vi "UHR-Fleezers Control (host) - Lorentz v4.vi"() -> ()   [LabVIEW 2014] (continued)
                n2998 = call "move to saved stage position.vi"("Stage VISA resource name in"=w4451, "Position"=3, "Saved Stage Positions"=w4454) -> ("error out"=w4453:errorcluster)  [unwired: 1 in, 1 out]
                n2999 = local write "Stage Control Serial Error"(w4453) -> ()
              }
              frame #5 {
                w4456 = FALSE ("Stage Moving")
                n3000 = local write "Stage Moving"(w4456) -> ()
                n3001 = local write "AL Running"(w4456) -> ()
                n3002 = call <vilib>:"Beep.vi"() -> ()  [unwired: 3 in, 9 out]
              }
            }
          }
        }
      }
      event "Stop All": Value Change {
        n3003 = event-data() -> ()  [unwired: 7 out]
        n3004 = local read "Stop All"() -> (w4457:bool)
      }
    }
    n3005 = node-c288() -> ()  [unwired: 2 out]
  }
  n3006 = node-c288(w50) -> ()  [unwired: 1 out]
  n3007 = node-c288(w82) -> ()  [unwired: 1 out]
  n3008 = node-c288(w84) -> ()  [unwired: 1 out]
  n3009 = node-c288(w72) -> ()  [unwired: 1 out]
  n3010 = property on="Saved trap pos" class="WFGraph (strict)"("Visible"=FALSE) -> ()  [unwired: 2 in, 2 out]
  n3011 = property on="Trap Delta Graph" class="WFGraph (strict)"("Visible"=TRUE) -> ()  [unwired: 2 in, 2 out]
  n3012 = disable-structure shown="Disabled" {
    disable-tunnel: w75 -> [w4459 _]
    disable-tunnel: w74 -> [w4458 _]
    frame Disabled {
      n3013 = VISA Close(VISA resource name=w4459, error in (no error)=w4458) -> (error out=w4460:errorcluster)
      n3014 = call <vilib>:"Simple Error Handler.vi"("error in (no error)"=w4460) -> ()  [unwired: 1 in, 8 out]
    }
    frame Enabled {
    }
  }
  n3015 = disable-structure shown="Disabled" {
    disable-tunnel: [w4468 _] -> w36
    disable-tunnel: [w4464 _] -> w35
    disable-tunnel: [w4463 _] -> w34
    disable-tunnel: [w4462 _] -> w33
    disable-tunnel: [w4461 _] -> w32
    frame Disabled {
      # "n samples needed for data"
      n3016 = Unbundle By Name("sound format") -> ("sample rate (S/s)"=w4464:dbl)
      n3017 = call <vilib>:"Sound Output Configure.vi"("number of samples/ch"="number of samples/ch", "sample mode"="sample mode", "sound format"="sound format", "device ID"="device ID") -> ("task ID"=w4468:T60)  [unwired: 6 in, 1 out]
      n3018 = local read "DMA Update Period (s)"() -> (w4465:dbl)
      n3019 = Multiply(x=w4465, y=w4464) -> (x*y=w4463:dbl)
      n3020 = for "Sound time base" {
        N: w4463 -> [_]
        tunnel: [w4472] -> w4466 mode=indexing
        i -> [w4472]
      }
      n3021 = Reciprocal(x=w4464) -> (1/x=w4462:dbl)
      n3022 = Multiply(x=w4466, y=w4462) -> (x*y=w4461:dbl[])
    }
    frame Enabled {
    }
  }
  n3023 = timed-loop "Main data acquisition loop (get data, process data for display, and save data to disk)" {
    tunnel: w31 -> [w4562]
    tunnel: w44 -> [w4561]
    tunnel: [w4821] -> w96
    tunnel: [w4816] -> w95
    timing: w89 -> [_]
    timing-out: [_] -> w88
    tunnel: w66 -> [w4728]
    tunnel: [w4618] -> w37
    tunnel: w36 -> [w4617]
    tunnel: w35 -> [w4615]
    tunnel: w34 -> [w4614]
    tunnel: w33 -> [w4613]
    tunnel: w32 -> [w4612]
    tunnel: w21 -> [w4553]
    tunnel: w20 -> [w4552]
    tunnel: [w4547] -> w19
    stop <- "Stop All" stop-if-true
    w4492 = 2.0
    w4518 = 3276.7
    w4675 = "Initialize"
    # "Cursor control of MCL trap position"
    # "Values for plotting"
    # "Added by Ronen - the limits imposed on amplitudes sent to AOM\nare not explicitly imposed when using intensity feedback. At amplitude of \n~48% FB intensity is ~1.8, if while feedback is on the value passes 1.8, feedback\nis turned off (indication that feedback algorithm overshoots)."
    # "List of channels in order (X or Y only):\nT1 X (mV)\nT2 X (mV)\nT1 X (nm)\nT2 X (nm)\nT1 FX (pN)\nT2 FX (pN)\nPosition Difference (nm)\nAPD1\nAPD2\nAPD3"
    # "T2 sum"
    # "T1 sum"
    n3024 = node-c288() -> ()  [unwired: 2 out]
    n3025 = First Call?() -> (First Call?: T/F=w4688:bool)
    n3026 = Or(x="Reset", y=w4688) -> (x .or. y?=w4689:bool)
    n3027 = Or(x="Start AOD Scan", y="Trap Raster Scan") -> (x .or. y?=w4775:bool)
    n3028 = case "Reset data stream (manual reset or at begining of some rastering and imaging)" shown="True" w4689 {
      tunnel: w4562 -> [w5574 w5582]
      tunnel: w4561 -> [w5573 w5581]
      tunnel: [w5574 w5576] -> w4592
      tunnel: [w5573 w5575] -> w4593
      frame False {
      }
      frame True {
        w5579 = TRUE ("AI to FIFO")
        n3029 = call "reset FPGA DMA.vi"("error in"=w5581, "FPGA VI Reference In"=w5582) -> ("error out"=w5577:errorcluster, "FPGA VI Reference Out"=w5578:T50)
        n3030 = local write "Overflow (data lost)"(FALSE ("Overflow (data lost)")) -> ()
        n3031 = xnode "Read/Write Control"("FPGA VI Reference In"=w5578, "error in"=w5577, "AI to FIFO"=w5579, "APD to FIFO"=w5579) -> ("FPGA VI Reference Out"=w5576:T50, "error out"=w5575:errorcluster)
      }
    }
    n3032 = case "Start active calibration (oscillate traps precisely)" shown="True" "Active Cal" {
      tunnel: w4593 -> [w4924 w4932]
      tunnel: w4592 -> [w4923 w4933]
      tunnel: [w4924 w4929] -> w4591
      tunnel: [w4923 w4930] -> w4590
      frame False {
      }
      frame True {
        w4925 = TRUE ("APD to FIFO")
        n3033 = call "reset FPGA DMA.vi"("error in"=w4932, "FPGA VI Reference In"=w4933) -> ("error out"=w4926:errorcluster, "FPGA VI Reference Out"=w4927:T50)
        n3034 = local write "Active Cal"(FALSE ("Active Cal")) -> ()
        n3035 = local write "Save Calibration"(TRUE ("Save Calibration")) -> ()
        n3036 = xnode "Read/Write Control"("FPGA VI Reference In"=w4927, "error in"=w4926, "AI to FIFO"=w4925, "APD to FIFO"=w4925) -> ("FPGA VI Reference Out"=w4930:T50, "error out"=w4929:errorcluster)
      }
    }
    n3037 = case shown="True" "Read Lateness and Rel Phase" {
      tunnel: w4562 -> [w5148 w5179]
      tunnel: w4561 -> [w5149 w5178]
      tunnel: [w5148 w5150] -> w4514
      tunnel: [w5149 w5151] -> w4764
      frame False {
      }
      frame True {
        n3038 = xnode "Read/Write Control"("FPGA VI Reference In"=w5179, "error in"=w5178) -> ("FPGA VI Reference Out"=w5150:T50, "error out"=w5151:errorcluster, "GI Relative phase"=→"GI relative phase":i16, "Relative phase"=→"Relative phase (AI1)":i16, "AI Late Counter"=→"Late Counter (AI1)":u8, "GI Late Counter"=→"GI Late Counter":u8, "MCL Late Counter"=→"MCL Late Counter":u8, "MCL Relative Phase"=→"Relative Phase (MCL)":i16, "APD Acq Relative Phase"=→"APD Acq Relative Phase":i16, "APD 1 Gate Relative Phase"=→"APD 1 Gate Relative Phase":i16, "APD 2 Gate Relative Phase"=→"APD 2 Gate Relative Phase":i16, "APD Acq Late Counter"=→"APD Acq Late Counter":u8, "APD 1 Gate Late Counter"=→"APD 1 Gate Late Counter":u8, "APD 2 Gate Late Counter"=→"APD 2 Gate Late Counter":u8, "Green FB Relative Phase"=→"Relative phase (Green FB)":i16, "GI Relative phase 2"=→"GI relative phase 2":i16, "GI Late Counter 2"=→"GI Late Counter 2":u8, "Trap Pos FIFO Timeout"=→"Trap Pos FIFO Timeout":u16, "Trap AI FIFO Timeout"=→"Trap AI FIFO Timeout":u16, "RI Late Counter"=→"RI Late Counter":u8, "RI Relative phase"=→"RI relative phase":i16, "Green Late Counter"=→"Green AI Late Counter":u8, "BI Late Counter (AO)"=→"Late Counter (BI AO)":u8, "Blue Late Counter (D)"=→"Late Counter (BI DO)":u8, "BI Relative phase (AO)"=→"Relative phase (BI AO)":i16, "BI Relative phase (D)"=→"Relative phase (BI DO)":i16, "APD 3 Gate Late Counter"=→"APD 3 Gate Late Counter":u8, "APD 3 Gate Relative Phase"=→"APD 3 Gate Relative Phase":i16)
      }
    }
    n3039 = Compound Arithmetic op=OR("Start MCL Scan", "Confocal Image", "Confocal Linescan") -> (w4560:bool)
    n3040 = And(x="Save Data (MCL)", y=w4560) -> (x .and. y?=w4794:bool)
    n3041 = case "Start AOM raster scan" shown="True" w4775 {
      tunnel: w4590 -> [w5433 w5443]
      tunnel: w4591 -> [w5432 w5442]
      tunnel: [w5433 w5436] -> w4797
      tunnel: [w5432 w5435] -> w4796
      frame False {
      }
      frame True {
        n3042 = case shown="True" "Restart DMA? (AOD)" {
          tunnel: [w5472 w5474] -> w5437
          tunnel: [w5471 w5473] -> w5438
          tunnel: w5443 -> [w5472 w5476]
          tunnel: w5442 -> [w5471 w5475]
          frame False {
          }
          frame True {
            n3043 = local write "Overflow (data lost)"(FALSE ("Overflow (data lost)")) -> ()
            n3044 = call "reset FPGA DMA.vi"("error in"=w5475, "FPGA VI Reference In"=w5476) -> ("error out"=w5473:errorcluster, "FPGA VI Reference Out"=w5474:T50)
          }
        }
        n3045 = local write "Trap Raster Scan"(FALSE ("Trap Raster Scan")) -> ()
        n3046 = case shown="True" "Move MCL Also?" {
          tunnel: w5438 -> [w5446 w5466]
          tunnel: w5437 -> [w5447 w5467]
          tunnel: [w5445 w5470] -> w5436
          tunnel: [w5444 w5469] -> w5435
          frame False {
            w5448 = TRUE ("AI to FIFO")
            n3047 = xnode "Read/Write Control"("FPGA VI Reference In"=w5447, "error in"=w5446, "AI to FIFO"=w5448, "APD to FIFO"=w5448, "Start scan"=w5448) -> ("FPGA VI Reference Out"=w5445:T50, "error out"=w5444:errorcluster)
          }
          frame True {
            w5464 = FALSE ("1D or 2D Scan?")
            w5468 = TRUE ("AI to FIFO")
            n3048 = local read "Scan Range (nm)"() -> (w5461:dbl)
            n3049 = local read "Scan steps (AOD)"() -> (w5455:u64)
            n3050 = local read "Total Counts (ticks)"() -> (w5456:u16)
            n3051 = local read "Cycles/step (AOD)"() -> (w5454:u64)
            n3052 = local read "Number of F/B Scans (AOD)"() -> (w5463:u16)
            n3053 = Bundle("Scan Range (nm)"=w5461, "MCL Step Position Ratio"="MCL Step Position Ratio", "MCL/AOM Scale Tweak"="MCL/AOM Scale Tweak", "MCL X Cal (nm/V)"="MCL X Cal (nm/V)", "MCL Step Increment (V_int)"="MCL Step Increment (V_int)", "Total Counts (ticks)"=w5456, "Scan steps (AOD)"=w5455, "Cycles/step (AOD)"=w5454) -> (w5453:T67)  [unwired: 1 in]
            n3054 = call "Calculate MCL scan parameters.vi"("Input parameters"=w5453) -> ("Scan steps(MCL)"=w5452:dbl, "Scan Freq. Increment (MCL)"=w5451:dbl, "MCL Count"=w5450:dbl)
            "MCL Count" <- w5450
            n3055 = xnode "Read/Write Control"("FPGA VI Reference In"=w5467, "error in"=w5466, "Scan steps (MCL)"=w5452, "Number of scans (MCL)"=w5463, "Cycles per step (MCL)"=u64 1, "Scan freq.  increment (MCL)"=w5451, "1D or 2D Scan?"=w5464, "MCL Scan Axis"=w5464, "Cont. Scan (MCL)"=w5464, "MCL count"=w5450) -> ("FPGA VI Reference Out"=w5449:T50, "error out"=w5465:errorcluster)
            n3056 = local write "MCL Scanning"(w5468) -> ()
            n3057 = local write "wait to reset values"(w5468) -> ()
            n3058 = xnode "Read/Write Control"("FPGA VI Reference In"=w5449, "error in"=w5465, "AI to FIFO"=w5468, "APD to FIFO"=w5468, "Start scan"=w5468, "Start scan (MCL)"=w5468) -> ("FPGA VI Reference Out"=w5470:T50, "error out"=w5469:errorcluster)
          }
        }
        "Raster Scanning..." <- TRUE ("Scanning...")
      }
    }
    n3059 = case "Start MCL raster scan" shown="True" w4560 {
      tunnel: w4797 -> [w5361 w5376]
      tunnel: w4796 -> [w5360 w5375]
      tunnel: [w5361 w5371] -> w4727
      tunnel: [w5360 w5370] -> w4726
      tunnel: [FALSE w5369] -> w4780
      tunnel: "Start MCL Scan" -> [_ w5364]
      tunnel: "Confocal Image" -> [_ w5363]
      tunnel: "Confocal Linescan" -> [_ _]
      frame False {
      }
      frame True {
        w5369 = TRUE
        n3060 = case shown="True" "Restart DMA? (MCL)" {
          tunnel: [w5405 w5407] -> w5374
          tunnel: [w5404 w5406] -> w5373
          tunnel: w5376 -> [w5405 w5410]
          tunnel: w5375 -> [w5404 w5409]
          frame False {
          }
          frame True {
            n3061 = call "reset FPGA DMA.vi"("error in"=w5409, "FPGA VI Reference In"=w5410) -> ("error out"=w5406:errorcluster, "FPGA VI Reference Out"=w5407:T50)
            n3062 = local write "Overflow (data lost)"(FALSE ("Overflow (data lost)")) -> ()
          }
        }
        n3063 = case shown="False" w5364 {
          tunnel: w5363 -> [w5379 _]
          frame False {
            n3064 = property on="Confocal Image" class="Bool (strict)"("Value"=FALSE ("Start Confocal Map")) -> ()  [unwired: 2 in, 2 out]
            n3065 = property on="2D or 1D Scan" class="Bool (strict)"("Val(Sgnl)"=w5379) -> ()  [unwired: 2 in, 2 out]
          }
          frame True {
          }
        }
        n3066 = local write "Tab Control 6"(T4."Imaging" ("Tab Control 6")) -> ()
        n3067 = local write "MCL Scanning"(w5369) -> ()
        n3068 = local read "AO2"() -> (w5365:dbl)
        n3069 = local read "AO1"() -> (w5366:dbl)
        n3070 = case shown="True" "Center Scan" {
          tunnel: w5374 -> [w5386 w5403]
          tunnel: w5373 -> [w5385 w5402]
          tunnel: [w5384 w5401] -> w5371
          tunnel: [w5383 w5400] -> w5370
          tunnel: [w5381 w5388] -> w5368
          tunnel: [w5380 w5387] -> w5367
          tunnel: w5366 -> [w5381 w5393]
          tunnel: w5365 -> [w5380 w5392]
          frame False {
            w5382 = TRUE ("AI to FIFO")
            n3071 = xnode "Read/Write Control"("FPGA VI Reference In"=w5386, "error in"=w5385, "AI to FIFO"=w5382, "APD to FIFO"=w5382, "Start scan (MCL)"=w5382) -> ("FPGA VI Reference Out"=w5384:T50, "error out"=w5383:errorcluster)
          }
          frame True {
            w5399 = TRUE ("AI to FIFO")
            n3072 = local read "Actual MCL Inc (V)"() -> (w5396:dbl)
            n3073 = local read "Scan steps (MCL)"() -> (w5395:u64)
            n3074 = local read "Scan lines (y)"() -> (w5394:u64)
            n3075 = local read "2D or 1D Scan"() -> (w5389:bool)
            n3076 = local read "Fast Scan Dir"() -> (w5390:bool)
            n3077 = Bundle("Actual MCL Inc (V)"=w5396, "Scan steps (MCL)"=w5395, "Scan lines (y)"=w5394, "AO1"=w5393, "AO2"=w5392) -> (w5391:T68)  [unwired: 1 in]
            n3078 = call "Center Scan calculation.vi"("2D or 1D Scan"=w5389, "Fast Scan Dir"=w5390, "Input parameters"=w5391) -> ("AO2"=w5387:dbl, "AO1"=w5388:dbl)
            n3079 = call "Volt to I16.vi"("Voltage In"=w5388) -> ("I16 Voltage Out"=w5398:i16)
            n3080 = call "Volt to I16.vi"("Voltage In"=w5387) -> ("I16 Voltage Out"=w5397:i16)
            n3081 = xnode "Read/Write Control"("FPGA VI Reference In"=w5403, "error in"=w5402, "AI to FIFO"=w5399, "APD to FIFO"=w5399, "Start scan (MCL)"=w5399, "AO1"=w5398, "AO2"=w5397) -> ("FPGA VI Reference Out"=w5401:T50, "error out"=w5400:errorcluster)
          }
        }
        "Initial Y" <- w5368
        "Initial X" <- w5367
        "wait to reset values" <- w5369
      }
    }
    n3082 = xnode "Read/Write Control"("FPGA VI Reference In"=w4514) -> ("FPGA VI Reference Out"=w4473:T50, "BD1 Frequency Out 1"=w4516:u64)  [unwired: 1 in, 1 out]
    n3083 = And(x="Save scans", y=w4775) -> (x .and. y?=w4795:bool)
    n3084 = call "IR AOM word to freq.vi"("Frequency Word In (U64)"=w4516) -> ("Frequency Out (MHz)"=w4515:dbl)
    n3085 = local read "BD 1 Frequency 2 (MHz)"() -> (w4575:dbl)
    n3086 = Subtract(x=w4575, y=w4515) -> (x-y=w4568:dbl)
    "Current deltaF (MHz)" <- w4568
    n3087 = control-ref of="Piezo trap cursor control"() -> (w4474:refnum<vi>)
    n3088 = Unbundle By Name("Cursor control") -> ("X"=w4476:bool, "Y"=w4475:bool)
    n3089 = local read "APD Elements/DMA read"() -> (w4632:u32)
    n3090 = local read "Trap AI Elements/DMA read"() -> (w4762:u32)
    n3091 = case shown="False" w4476 {
      tunnel: w4474 -> [w4848 w4858]
      tunnel: w4473 -> [_ w4850]
      frame False {
        n3092 = local read "T3 X (V)"() -> (w4849:dbl)
        n3093 = property class="XYGraph (strict)"(reference=w4848, "Cursor.Cursor X"=w4849) -> ()  [unwired: 1 in, 2 out]
      }
      frame True {
        n3094 = property class="XYGraph (strict)"(reference=w4858) -> ("Cursor.Cursor X"=w4855:dbl)  [unwired: 1 in, 2 out]
        n3095 = In Range and Coerce(upper limit=10.0, x=w4855, lower limit=0.0) -> (coerced(x)=w4853:dbl)  [unwired: 1 out]
        n3096 = Multiply(x=3276.7, y=w4853) -> (x*y=w4852:dbl)
        n3097 = To Unsigned Word Integer(number=w4852) -> (unsigned 16bit integer=w4851:u16)
        n3098 = xnode "Read/Write Control"("FPGA VI Reference In"=w4850, "Piezo Trap X (AO5)"=w4851) -> ()  [unwired: 1 in, 2 out]
      }
    }
    n3099 = case shown="False" w4475 {
      tunnel: w4474 -> [w4835 w4847]
      tunnel: w4473 -> [_ w4838]
      frame False {
        n3100 = local read "T3 Y (V)"() -> (w4837:dbl)
        n3101 = Negate(x=w4837) -> (-x=w4836:dbl)
        n3102 = property class="XYGraph (strict)"(reference=w4835, "Cursor.Cursor Y"=w4836) -> ()  [unwired: 1 in, 2 out]
      }
      frame True {
        n3103 = property class="XYGraph (strict)"(reference=w4847) -> ("Cursor.Cursor Y"=w4844:dbl)  [unwired: 1 in, 2 out]
        n3104 = In Range and Coerce(upper limit=0.0, x=w4844, lower limit=-10.0) -> (coerced(x)=w4843:dbl)  [unwired: 1 out]
        n3105 = Negate(x=w4843) -> (-x=w4841:dbl)
        n3106 = Multiply(x=3276.7, y=w4841) -> (x*y=w4840:dbl)
        n3107 = To Unsigned Word Integer(number=w4840) -> (unsigned 16bit integer=w4839:u16)
        n3108 = xnode "Read/Write Control"("FPGA VI Reference In"=w4838, "Piezo Trap Y (AO4)"=w4839) -> ()  [unwired: 1 in, 2 out]
      }
    }
    n3109 = local read "Trap Pos Elements/DMA read"() -> (w4723:u32)
    n3110 = local read "DMA Update Period (s)"() -> (w4550:dbl)
    n3111 = xnode "Invoke Method"("FPGA VI Reference In"=w4727, "error in"=w4726, "Number of Elements"=w4723, "Timeout (ms)"=-1) -> ("Data"=w4695:u16[], "Elements Remaining"=→"Trap Pos FIFO El Remaining":u32)  [unwired: 2 out]
    n3112 = xnode "Get Trap Data"("FPGA VI Reference In"=w4727, "error in"=w4726, "Number of Elements"=w4762, "Timeout (ms)"=-1 ("Timeout")) -> ("FPGA VI Reference Out"=w4574:T50, "error out"=w4665:errorcluster, "Data"=w4557:i16[], "Elements Remaining"=w4829:u32)
    "FIFO El. Rem." <- w4829
    n3113 = local read "Trap AI FIFO Depth"() -> (w4831:u32)
    n3114 = xnode "Get APD Data"("FPGA VI Reference In"=w4727, "error in"=w4726, "Number of Elements"=w4632, "Timeout (ms)"=-1) -> ("Data"=w4529:u32[], "Elements Remaining"=→"APD FIFO Elements Remaining":u32)  [unwired: 2 out]
    n3115 = feedback #1(0.0) -> (w4718:dbl)
    n3116 = To Time Stamp(1:w4718) -> (0:w4512:timestamp)
    n3117 = Add(x=w4550, y=w4718) -> (x+y=w4806:dbl)
    n3118 = feedback-in #1(w4806) -> ()
    n3119 = Subtract(x=w4831, y=w4762) -> (x-y=w4830:u32)
    n3120 = local read "APD Integration Time (s)"() -> (w4521:dbl)
    n3121 = Divide(x=w4829, y=w4830) -> (x/y=w4828:dbl)
    "Buffer Status" <- w4828
    n3122 = local read "Trap Sets"() -> (w4558:u32)
    n3123 = Divide(x=w4550, y="PSD Data Period (s)") -> (x/y=w4549:dbl)
    n3124 = Equal?(x=w4828, y=1.0) -> (x = y?=w4826:bool)
    n3125 = local read "Number of APDs"() -> (w4528:u8)
    n3126 = Decimate 1D Array(w4695) -> (w4692:u16[], w4694:u16[], w4693:u16[], w4519:u16[], w4517:u16[])
    n3127 = To Unsigned Long Integer(number=w4549) -> (unsigned 32bit integer=w4548:u32)
    n3128 = case "Alert buffer overflow" shown="True" w4826 {
      frame False {
      }
      frame True {
        n3129 = call <vilib>:"Beep.vi"() -> ()  [unwired: 3 in, 9 out]
        "Overflow (data lost)" <- TRUE ("Overflow (data lost)")
      }
    }
    n3130 = To Unsigned Long Integer(number=w4692) -> (unsigned 32bit integer=w4691:u32[])
    n3131 = Join Numbers(hi=w4694, lo=w4693) -> ((hi.lo)=w4690:u32[])
    n3132 = Divide(x=w4519, y=w4518) -> (x/y=w4500:dbl[])
    n3133 = Divide(x=w4517, y=w4518) -> (x/y=w4499:dbl[])
    n3134 = call "Arduino input-output.vi"("VISA resource name"=w4553, "Sets to read"=w4548, "Error in"=w4552) -> ("VISA resource out"=w4547:refnum<visa-resource-name>, "Channel names"=w4537:string[], "Output"=w4536:dbl[][], "Error out"=→"Serial Error out":errorcluster)
    n3135 = call "deinterlace.vi"("Detector type"="Detector Type", "Data"=w4557, "Trap sets"=w4558, "Flip x sign"="Flip X Sign") -> ("Channel pattern"=w4554:i32, "Channel names"=w4533:string[], "Deinterlaced normalized data"=w4534:dbl[][], "Deinterlaced data"=w4555:i16[])
    n3136 = Join Numbers(hi=w4691, lo=w4690) -> ((hi.lo)=w4685:u64[])
    n3137 = local read "Data Period (s)"() -> (w4506:dbl)
    n3138 = call "APD data extraction.vi"("Data"=w4529, "Number of APD's"=w4528, "APD integration time (s)"=w4521, "APD Ave N"="APD Ave N", "APD Disp. Downsample"="APD Disp. Downsample", "APD Disp. Scale"="APD Disp. Scale", "Time Stamp"=w4512) -> ("Output cluster"=→"APD rates cluster":T2, "Output Data"=w4524:T69, "Output waveform"=w4523:waveform(dbl)[], "APD Display period (s)"=w4522:dbl)
    "APD Display Period (s)" <- w4522
    n3139 = call "IR AOM word to freq - vec.vi"("Frequency Word In (double vec)"=w4685) -> ("Frequency Out"=w4722:dbl[])
    n3140 = Decimate 1D Array(w4499) -> (w4496:dbl[], w4495:dbl[])
    n3141 = Decimate 1D Array(w4500) -> (w4498:dbl[], w4497:dbl[])
    n3142 = Add(x=w4498, y=w4497) -> (x+y=w4494:dbl[])
    n3143 = Add(x=w4496, y=w4495) -> (x+y=w4493:dbl[])
    n3144 = Decimate 1D Array(w4722) -> (w4721:dbl[], w4720:dbl[])
    n3145 = Divide(x=w4494, y=w4492) -> (x/y=w4490:dbl[])
    n3146 = Divide(x=w4493, y=w4492) -> (x/y=w4491:dbl[])
    n3147 = Reciprocal(x=w4522) -> (1/x=→"APD Display Freq. (Hz)":dbl)
    n3148 = call "Generate Waveform.vi"("Downsampling"="PSD downsample", "Data Period (s)"="PSD Data Period (s)", "Data"=w4536, "Plot names"=w4537, "Time Stamp"=w4512) -> ("Downsampled data"=w4535:waveform(dbl)[])  [unwired: 1 out]
    n3149 = Build Array(w4721, w4720, w4490, w4491) -> (w4513:dbl[][])
    n3150 = for {
      tunnel: w4536 -> [w4874] mode=indexing
      tunnel: [w4873] -> w4543 mode=indexing
      n3151 = call-poly <vilib>:"Mean.vi"("X"=w4874) -> ("mean"=w4873:dbl)  [unwired: 1 out]
    }
    n3152 = Multiply(x=w4506, y="Trap Disp. Downsample") -> (x*y=w4719:dbl)
    "Display Period (s)" <- w4719
    n3153 = for {
      tunnel: w4534 -> [w4876] mode=indexing
      tunnel: [w4875] -> w4542 mode=indexing
      n3154 = call-poly <vilib>:"Mean.vi"("X"=w4876) -> ("mean"=w4875:dbl)  [unwired: 1 out]
    }
    n3155 = call "Generate Waveform.vi"("Downsampling"="Trap Disp. Downsample", "Data Period (s)"=w4506, "Data"=w4534, "Plot names"=w4533, "Time Stamp"=w4512) -> ("Downsampled data"=w4531:waveform(dbl)[], "Non downsampled waveform"=w4530:waveform(dbl)[])
    n3156 = Multiply(x="APD Disp. Scale", y=w4523) -> (x*y=w4740:waveform(dbl)[])
    n3157 = Reciprocal(x=w4719) -> (1/x=→"Trap Disp. Freq. (Hz)":dbl)
    n3158 = Insert Into Array(array=w4543, index=0, new element=w4542) -> (→"Values":dbl[])
    n3159 = Multiply(x="APD Disp. Downsample", y=w4521) -> (x*y=w4739:dbl)
    n3160 = Decimate 1D Array(w4555) -> (w4710:i16[], w4709:i16[], w4707:i16[], w4706:i16[])  [unwired: 9 out]
    n3161 = Divide(x=w4740, y=w4739) -> (x/y=w4637:waveform(dbl)[])
    n3162 = Insert Into Array(array=w4537, index=0, new element=w4533) -> (→"AI labels":string[])
    n3163 = case shown="1" "Plot Trap Positions" {
      tunnel: [w4859 w4868] -> w4507
      frame 0, Default {
        n3164 = local read "BD 1 Frequency 2 (MHz)"() -> (w4862:dbl)
        n3165 = local read "BD 1 Frequency 1 (MHz)"() -> (w4863:dbl)
        n3166 = local read "T3 Y (V)"() -> (w4860:dbl)
        n3167 = local read "T3 X (V)"() -> (w4861:dbl)
        n3168 = Build Array(w4863, w4862, w4861, w4860) -> (w4859:dbl[])
      }
      frame 1 {
        w4867 = 75.0
        n3169 = Unbundle By Name("Piezo trap 0 position relative to 75 MHz") -> ("X (V)"=w4865:dbl, "Y (V)"=w4864:dbl)
        n3170 = Build Array(w4867, w4867, w4865, w4864) -> (w4868:dbl[])
      }
    }
    n3171 = Divide(x=w4710, y=w4709) -> (x/y=w4711:dbl[])
    n3172 = Divide(x=w4707, y=w4706) -> (x/y=w4708:dbl[])
    n3173 = local read "AOM X Cal (nm/MHz)"() -> (w4509:dbl)
    n3174 = Split 1D Array(array=w4711, index="N El. to Ave.") -> (second subarray=w4714:dbl[])  [unwired: 1 out]
    n3175 = Split 1D Array(array=w4708, index="N El. to Ave.") -> (second subarray=w4713:dbl[])  [unwired: 1 out]
    n3176 = Index Array(array=w4637, index=0) -> (element=w4735:waveform(dbl))
    n3177 = Index Array(array=w4637, index=1) -> (element=w4733:waveform(dbl))
    n3178 = Index Array(array=w4637, index=2) -> (element=w4639:waveform(dbl))
    n3179 = call-poly <vilib>:"Mean.vi"("X"=w4714) -> ("mean"=w4702:dbl)  [unwired: 1 out]
    n3180 = call-poly <vilib>:"Mean.vi"("X"=w4713) -> ("mean"=w4701:dbl)  [unwired: 1 out]
    n3181 = Subtract(x=w4735, y="APD 1 Offset") -> (x-y=w4731:waveform(dbl))
    n3182 = Subtract(x=w4733, y="APD 2 Offset") -> (x-y=w4730:waveform(dbl))
    n3183 = Subtract(x=w4639, y="APD 3 Offset") -> (x-y=w4636:waveform(dbl))
    n3184 = Build Array(w4731, w4730, w4636) -> (→"APD Chart":waveform(dbl)[])
    n3185 = Build Array(w4509, w4509, "Piezo Trap X cal (nm/V)", "Piezo Trap Y cal (nm/V)") -> (w4508:dbl[])
    n3186 = local read "Trap X AI1 (DMA)"() -> (w4712:T19)
    n3187 = To Fixed-Point(number=w4701) -> (fixed-point=w4699:fxp<+/-,16,1>)  [unwired: 1 in]
    n3188 = To Fixed-Point(number=w4702) -> (fixed-point=w4700:fxp<+/-,16,1>)  [unwired: 1 in]
    n3189 = Cluster To Array(cluster="Negate Axis") -> (array=w4501:bool[])
    n3190 = call "Generate Trap Positiion Waveform.vi"("Base trap positions"=w4507, "Data Period (s)"=w4506, "Input data"=w4513, "Position calibration values"=w4508, "Trap Pos. Disp. Downsample (s)"="Trap Pos. Disp. Downsample", "Negate axis"=w4501, "Time Stamp"=w4512) -> ("Output waveforms"=w4478:waveform(dbl)[])  [unwired: 3 in]
    "Trap Positions" <- w4478
    n3191 = Bundle By Name(cluster=w4712, "Set 1"=w4700, "Set 2"=w4699) -> (→"Trap X AI1 (DMA)":T19)
    n3192 = Initialize Array(0.0) -> (w4503:dbl[][])  [unwired: 2 in]
    n3193 = local read "Display Period (s)"() -> (w4749:dbl)
    n3194 = for {
      tunnel: w4478 -> [w4872] mode=indexing
      shift-right: [w4870] -> w4480
      shift-left: w4503 -> [w4871]
      n3195 = Unbundle By Name(w4872) -> ("Y"=w4869:dbl[])
      n3196 = Build Array (concatenate)(w4871, w4869) -> (w4870:dbl[][])
    }
    n3197 = Build Array (concatenate)(w4523, w4531, w4535) -> (w4544:waveform(dbl)[])
    "All Signals" <- w4544
    n3198 = Divide(x="Bead Sep. Int. Time (s)", y=w4749) -> (x/y=w4486:dbl)
    n3199 = feedback #2(w4480) -> (w4487:dbl[][])
    n3200 = call "Trap Pos RMS.vi"("Accumulated array"=w4487, "New Array"=w4480, "Number of sets to average"=w4486) -> ("Output accumulated array"=w4485:dbl[][], "RMS"=w4483:dbl[], "Mean"=w4484:dbl[])
    n3201 = feedback-in #2(w4485) -> ()
    n3202 = Index Array(array=w4480, index (row)=0 ("index")) -> (element=w4479:dbl[])  [unwired: 1 in]
    n3203 = Array To Cluster(array=w4483) -> (cluster=→"Trap RMS (ang)":T70)
    n3204 = Array To Cluster(array=w4484) -> (cluster=→"Mean Trap Positions (nm)":T71)
    n3205 = local read "Data points/scans (MCL)"() -> (w4789:dbl)
    n3206 = Unbundle(w4524) -> ("APD 1"=w4635:u32[])  [unwired: 2 out]
    n3207 = To Double Precision Float(number=w4635) -> (double precision float=w4757:dbl[])
    n3208 = Increment(x=w4789) -> (x+1=w4790:dbl)
    n3209 = feedback #3(w4790) -> (w4793:dbl)
    n3210 = Select(t=0, s=w4780, f=w4793) -> (s? t:f=w4786:dbl)
    n3211 = Array Size(array=w4757) -> (size(s)=w4792:i32)
    n3212 = Add(x=w4792, y=w4786) -> (x+y=w4787:dbl)
    n3213 = Greater?(x=w4787, y=w4789) -> (0:w4788:bool)
    n3214 = Select(t=w4786, s=w4788, f=w4787) -> (s? t:f=w4785:dbl)
    n3215 = feedback-in #3(w4785) -> ()
    n3216 = local read "MCL Scanning"() -> (w4783:bool)
    n3217 = Index Array(array=w4531, index="index 1") -> (element=w4627:waveform(dbl))
    n3218 = Index Array(array=w4531, index="index 2") -> (element=w4631:waveform(dbl))
    n3219 = Unbundle By Name(w4627) -> ("Y"=w4626:dbl[])
    n3220 = Unbundle By Name(w4631) -> ("Y"=w4630:dbl[])
    n3221 = Not(x=w4788) -> (.not. x?=w4782:bool)
    n3222 = And(x=w4782, y=w4783) -> (x .and. y?=w4784:bool)
    n3223 = call-poly <vilib>:"Mean.vi"("X"=w4626) -> ("mean"=→"Trap 1 sum mean":dbl)  [unwired: 1 out]
    n3224 = call-poly <vilib>:"Mean.vi"("X"=w4630) -> ("mean"=→"Trap 2 sum mean":dbl)  [unwired: 1 out]
    n3225 = Or(x=w4784, y=w4780) -> (x .or. y?=w4781:bool)
    n3226 = Equal?(x="Tab Control 6", y=T61."High Res Display") -> (x = y?=w4759:bool)
    n3227 = case shown="True" "X or Y?" {
      tunnel: w4531 -> [w4985 w4991]
      tunnel: [w4986 w4990] -> w4601
      tunnel: [w4984 w4989] -> w4598
      frame False {
        n3228 = Index Array(array=w4985, index=0) -> (element=w4986:waveform(dbl))
        n3229 = Index Array(array=w4985, index=3) -> (element=w4984:waveform(dbl))
      }
      frame True {
        n3230 = Index Array(array=w4991, index=1) -> (element=w4990:waveform(dbl))
        n3231 = Index Array(array=w4991, index=4) -> (element=w4989:waveform(dbl))
      }
    }
    n3232 = case "For displaying the high resolution display (no downsampling)" shown="True" w4759 {
      tunnel: w4530 -> [_ w5124]
      frame False {
      }
      frame True {
        n3233 = Index Array(array=w5124, index="High Res. Display") -> (element=w5125:waveform(dbl))
        n3234 = call <vilib>:"Std Deviation and Variance.vi"("X"=w5125) -> ("mean"=w5132:dbl, "standard deviation"=w5137:dbl)  [unwired: 1 in, 1 out]
        "Mean Intensity" <- w5132
        "Sigma" <- w5137
        n3235 = Subtract(x=w5125, y=w5132) -> (x-y=w5131:waveform(dbl))
        n3236 = Select(t=w5131, s="Subtract mean", f=w5125) -> (s? t:f=→"1 Channel":waveform(dbl))
        n3237 = Divide(x=w5137, y=w5132) -> (x/y=→"Sigma/Mean":dbl)
        n3238 = feedback #4(1) -> (w5126:i32)
        n3239 = Greater Or Equal?(x=w5126, y="Slow mean N ave.") -> (x >= y?=w5139:bool)
        n3240 = Increment(x=w5126) -> (x+1=w5141:i32)
        n3241 = Select(t=1, s=w5139, f=w5141) -> (s? t:f=w5128:i32)
        n3242 = feedback-in #4(w5128) -> ()
        n3243 = feedback #5() -> (w5129:waveform(dbl))  [unwired: 1 out]
        n3244 = case shown="Default" w5126 {
          tunnel: [w5144 w5147] -> w5130
          tunnel: w5129 -> [w5146 _]
          tunnel: w5125 -> [w5145 w5147]
          frame Default {
            n3245 = call-poly <vilib>:"Append Waveforms.vi"("waveform B"=w5145, "waveform A"=w5146) -> ("waveform out"=w5144:waveform(dbl))  [unwired: 1 in, 8 out]
          }
          frame 1 {
          }
        }
        n3246 = feedback-in #5(w5130) -> ()
        n3247 = case shown="True" w5139 {
          tunnel: w5130 -> [_ w5143]
          frame False {
          }
          frame True {
            n3248 = call-poly <vilib>:"Mean.vi"("X"=w5143) -> ("mean"=→"Slow mean":dbl)  [unwired: 1 out]
          }
        }
      }
    }
    n3249 = case "For plotting results of scanning MCL (fluorescence and detection laser images)" shown="True" w4781 {
      tunnel: w4780 -> [_ w5225]
      tunnel: w4789 -> [_ _]
      tunnel: w4530 -> [_ w5321]
      tunnel: w4728 -> [_ w5253]
      tunnel: w4524 -> [_ w5231]
      frame False {
      }
      frame True {
        w5194 = u32 0 items=["Horizontal", "Vertical", "Central", "1st Diagonal", "2nd Diagonal"] ("Type of Symmetry")
        w5198 = u32 0 items=["Horizontal", "Vertical", "Central", "1st Diagonal", "2nd Diagonal"] ("Type of Symmetry")
        w5199 = u32 0 items=["Horizontal", "Vertical", "Central", "1st Diagonal", "2nd Diagonal"] ("Type of Symmetry")
        w5200 = u32 0 items=["Horizontal", "Vertical", "Central", "1st Diagonal", "2nd Diagonal"] ("Type of Symmetry")
        w5204 = u32 0 items=["Horizontal", "Vertical", "Central", "1st Diagonal", "2nd Diagonal"] ("Type of Symmetry")
        # "Modified by Ronen \nbecause we do not have\nthe license for the\ntwo last image \nmanipulation VI's"
        n3250 = Unbundle(w5231) -> ("APD 1"=w5230:u32[], "APD 2"=w5228:u32[], "APD 3"=w5226:u32[])
        n3251 = To Double Precision Float(number=w5230) -> (double precision float=w5229:dbl[])
        n3252 = To Double Precision Float(number=w5228) -> (double precision float=w5227:dbl[])
        n3253 = To Double Precision Float(number=w5226) -> (double precision float=w5219:dbl[])
        n3254 = Index Array(array=w5321, index=10) -> (element=w5327:waveform(dbl))
        n3255 = Index Array(array=w5321, index=11) -> (element=w5324:waveform(dbl))
        n3256 = local read "Cycles/step (MCL)"() -> (w5283:u64)
        n3257 = Index Array(array=w5321, index="Channel") -> (element=w5323:waveform(dbl))
        n3258 = Unbundle(w5253) -> ("New Image"=w5252:T1, "New Image"=w5251:T1, "New Image"=w5232:T1, "New Image"=w5233:T1, "New Image"=w5234:T1)
        n3259 = local read "Scan steps (MCL)"() -> (w5221:u64)
        n3260 = Unbundle By Name(w5327) -> ("Y"=w5285:dbl[])
        n3261 = Unbundle By Name(w5324) -> ("Y"=w5287:dbl[])
        n3262 = local read "Scan lines (y)"() -> (w5222:u64)
        n3263 = local read "N APD Samp/step"() -> (w5224:dbl)
        n3264 = Unbundle By Name(w5323) -> ("Y"=w5292:dbl[])
        n3265 = call "downsample 1D array - double.vi"("Ave N"=w5283, "Array In"=w5285) -> ("Array Out"=w5284:dbl[])  [unwired: 1 out]
        n3266 = call "downsample 1D array - double.vi"("Ave N"=w5283, "Array In"=w5287) -> ("Array Out"=w5286:dbl[])  [unwired: 1 out]
        n3267 = call "downsample 1D array - double.vi"("Ave N"=w5283, "Array In"=w5292) -> ("Array Out"=w5291:dbl[])  [unwired: 1 out]
        n3268 = Multiply(x=w5221, y=u64 2) -> (x*y=w5223:u64)
        n3269 = feedback #6(w5227) -> (w5271:dbl[])
        n3270 = Build Array (concatenate)(w5271, w5227) -> (w5270:dbl[])
        n3271 = feedback #7(w5219) -> (w5220:dbl[])
        n3272 = Build Array (concatenate)(w5220, w5219) -> (w5218:dbl[])
        n3273 = Select(t=w5227, s=w5225, f=w5270) -> (s? t:f=w5255:dbl[])
        n3274 = feedback-in #6(w5255) -> ()
        n3275 = Select(t=w5219, s=w5225, f=w5218) -> (s? t:f=w5236:dbl[])
        n3276 = feedback-in #7(w5236) -> ()
        n3277 = feedback #8(w5229) -> (w5346:dbl[])
        n3278 = Build Array (concatenate)(w5346, w5229) -> (w5329:dbl[])
        n3279 = Select(t=w5229, s=w5225, f=w5329) -> (s? t:f=w5333:dbl[])
        n3280 = feedback-in #8(w5333) -> ()
        n3281 = feedback #9(w5284) -> (w5335:dbl[])
        n3282 = Build Array (concatenate)(w5335, w5284) -> (w5326:dbl[])
        n3283 = feedback #10(w5291) -> (w5344:dbl[])
        n3284 = Build Array (concatenate)(w5344, w5291) -> (w5343:dbl[])
        n3285 = feedback #11(w5286) -> (w5337:dbl[])
        n3286 = Build Array (concatenate)(w5337, w5286) -> (w5338:dbl[])
        n3287 = Select(t=w5284, s=w5225, f=w5326) -> (s? t:f=w5288:dbl[])
        n3288 = feedback-in #9(w5288) -> ()
        n3289 = Select(t=w5291, s=w5225, f=w5343) -> (s? t:f=w5290:dbl[])
        n3290 = feedback-in #10(w5290) -> ()
        n3291 = Select(t=w5286, s=w5225, f=w5338) -> (s? t:f=w5289:dbl[])
        n3292 = feedback-in #11(w5289) -> ()
        n3293 = call "integrate 1D array interval - double.vi"("Ave N"=w5224, "Array In"=w5255) -> ("Array Out"=w5266:dbl[])  [unwired: 1 out]
        n3294 = call "integrate 1D array interval - double.vi"("Ave N"=w5224, "Array In"=w5236) -> ("Array Out"=w5247:dbl[])  [unwired: 1 out]
        n3295 = call "integrate 1D array interval - double.vi"("Ave N"=w5224, "Array In"=w5333) -> ("Array Out"=w5332:dbl[])  [unwired: 1 out]
        n3296 = Array Size(array=w5266) -> (size(s)=w5267:i32)
        n3297 = Array Size(array=w5247) -> (size(s)=w5248:i32)
        n3298 = Array Size(array=w5332) -> (size(s)=w5334:i32)
        n3299 = Multiply(x=w5222, y=w5223) -> (x*y=w5269:u64)
        n3300 = Multiply(x=w5222, y=w5223) -> (x*y=w5250:u64)
        n3301 = Multiply(x=w5222, y=w5223) -> (x*y=w5342:u64)
        n3302 = Subtract(x=w5269, y=w5267) -> (x-y=w5260:u64)
        n3303 = call-poly <vilib>:"Mean.vi"("X"=w5266) -> ("mean"=w5257:dbl)  [unwired: 1 out]
        n3304 = Subtract(x=w5250, y=w5248) -> (x-y=w5241:u64)
        n3305 = call-poly <vilib>:"Mean.vi"("X"=w5247) -> ("mean"=w5238:dbl)  [unwired: 1 out]
        n3306 = Subtract(x=w5342, y=w5334) -> (x-y=w5282:u64)
        n3307 = call-poly <vilib>:"Mean.vi"("X"=w5332) -> ("mean"=w5279:dbl)  [unwired: 1 out]
        n3308 = call-poly <vilib>:"Mean.vi"("X"=w5288) -> ("mean"=w5272:dbl)  [unwired: 1 out]
        n3309 = call-poly <vilib>:"Mean.vi"("X"=w5290) -> ("mean"=w5277:dbl)  [unwired: 1 out]
        n3310 = call-poly <vilib>:"Mean.vi"("X"=w5289) -> ("mean"=w5275:dbl)  [unwired: 1 out]
        n3311 = Initialize Array(1.0 ("element"), w5260) -> (w5256:dbl[])
        n3312 = Initialize Array(1.0 ("element"), w5241) -> (w5237:dbl[])
        n3313 = Initialize Array(1.0 ("element"), w5282) -> (w5273:dbl[])
        n3314 = Multiply(x=w5256, y=w5257) -> (x*y=w5258:dbl[])
        n3315 = Multiply(x=w5237, y=w5238) -> (x*y=w5239:dbl[])
        n3316 = Multiply(x=w5273, y=w5279) -> (x*y=w5280:dbl[])
        n3317 = Multiply(x=w5273, y=w5275) -> (x*y=w5276:dbl[])
        n3318 = Multiply(x=w5273, y=w5277) -> (x*y=w5278:dbl[])
        n3319 = Multiply(x=w5273, y=w5272) -> (x*y=w5274:dbl[])
        n3320 = Build Array (concatenate)(w5266, w5258) -> (w5268:dbl[])
        n3321 = Build Array (concatenate)(w5247, w5239) -> (w5249:dbl[])
        n3322 = Build Array (concatenate)(w5332, w5280) -> (w5341:dbl[])
        n3323 = Build Array (concatenate)(w5288, w5274) -> (w5336:dbl[])
        n3324 = Build Array (concatenate)(w5290, w5278) -> (w5340:dbl[])
        n3325 = Build Array (concatenate)(w5289, w5276) -> (w5339:dbl[])
        n3326 = Reshape Array(w5268, w5222, w5223) -> (w5264:dbl[][])
        n3327 = Reshape Array(w5249, w5222, w5223) -> (w5245:dbl[][])
        n3328 = Reshape Array(w5341, w5222, w5223) -> (w5319:dbl[][])
        n3329 = Reshape Array(w5336, w5222, w5223) -> (w5302:dbl[][])
        n3330 = Reshape Array(w5340, w5222, w5223) -> (w5294:dbl[][])
        n3331 = Reshape Array(w5339, w5222, w5223) -> (w5309:dbl[][])
        n3332 = Array Subset(array=w5264, index (col)=0 ("index"), length (col)=w5221) -> (w5263:dbl[][])  [unwired: 2 in]
        n3333 = Array Subset(array=w5264, index (col)=w5221) -> (w5261:dbl[][])  [unwired: 3 in]
        n3334 = Array Subset(array=w5245, index (col)=0 ("index"), length (col)=w5221) -> (w5244:dbl[][])  [unwired: 2 in]
        n3335 = Array Subset(array=w5245, index (col)=w5221) -> (w5242:dbl[][])  [unwired: 3 in]
        n3336 = Array Subset(array=w5309, index (col)=0 ("index"), length (col)=w5221) -> (w5314:dbl[][])  [unwired: 2 in]
        n3337 = Array Subset(array=w5309, index (col)=w5221) -> (w5312:dbl[][])  [unwired: 3 in]
        n3338 = Array Subset(array=w5319, index (col)=0 ("index"), length (col)=w5221) -> (w5318:dbl[][])  [unwired: 2 in]
        n3339 = Array Subset(array=w5319, index (col)=w5221) -> (w5316:dbl[][])  [unwired: 3 in]
        n3340 = Array Subset(array=w5294, index (col)=0 ("index"), length (col)=w5221) -> (w5300:dbl[][])  [unwired: 2 in]
        n3341 = Array Subset(array=w5294, index (col)=w5221) -> (w5298:dbl[][])  [unwired: 3 in]
        n3342 = Array Subset(array=w5302, index (col)=0 ("index"), length (col)=w5221) -> (w5307:dbl[][])  [unwired: 2 in]
        n3343 = Array Subset(array=w5302, index (col)=w5221) -> (w5305:dbl[][])  [unwired: 3 in]
        n3344 = for {
          tunnel: w5263 -> [w5350] mode=indexing
          tunnel: [w5349] -> w5262 mode=indexing
          workers-P: _ -> [_]
          n3345 = Reverse 1D Array(array=w5350) -> (reversed array=w5349:dbl[])
        }
        n3346 = for {
          tunnel: w5244 -> [w5348] mode=indexing
          tunnel: [w5347] -> w5243 mode=indexing
          workers-P: _ -> [_]
          n3347 = Reverse 1D Array(array=w5348) -> (reversed array=w5347:dbl[])
        }
        n3348 = for {
          tunnel: w5314 -> [w5356] mode=indexing
          tunnel: [w5355] -> w5313 mode=indexing
          workers-P: _ -> [_]
          n3349 = Reverse 1D Array(array=w5356) -> (reversed array=w5355:dbl[])
        }
        n3350 = for {
          tunnel: w5318 -> [w5358] mode=indexing
          tunnel: [w5357] -> w5317 mode=indexing
          workers-P: _ -> [_]
          n3351 = Reverse 1D Array(array=w5358) -> (reversed array=w5357:dbl[])
        }
        n3352 = for {
          tunnel: w5300 -> [w5352] mode=indexing
          tunnel: [w5351] -> w5299 mode=indexing
          workers-P: _ -> [_]
          n3353 = Reverse 1D Array(array=w5352) -> (reversed array=w5351:dbl[])
        }
        n3354 = for {
          tunnel: w5307 -> [w5354] mode=indexing
          tunnel: [w5353] -> w5306 mode=indexing
          workers-P: _ -> [_]
          n3355 = Reverse 1D Array(array=w5354) -> (reversed array=w5353:dbl[])
        }
        n3356 = Index Array(array=w5319, index (row)=0) -> (element=→"Waveform Graph":dbl[])  [unwired: 1 in]
        n3357 = Add(x=w5262, y=w5261) -> (x+y=w5254:dbl[][])
        n3358 = Add(x=w5243, y=w5242) -> (x+y=w5235:dbl[][])
        n3359 = Add(x=w5313, y=w5312) -> (x+y=w5311:dbl[][])
        n3360 = Add(x=w5317, y=w5316) -> (x+y=w5293:dbl[][])
        n3361 = Add(x=w5299, y=w5298) -> (x+y=w5297:dbl[][])
        n3362 = Add(x=w5306, y=w5305) -> (x+y=w5304:dbl[][])
        n3363 = Divide(x=w5297, y=2) -> (x/y=w5295:dbl[][])
        n3364 = Divide(x=w5311, y=2) -> (x/y=w5212:dbl[][])
        n3365 = To Single Precision Float(number=w5293) -> (single precision float=w5216:sgl[][])
        n3366 = To Single Precision Float(number=w5254) -> (single precision float=w5211:sgl[][])
        n3367 = To Single Precision Float(number=w5235) -> (single precision float=w5210:sgl[][])
        n3368 = Divide(x=w5304, y=2) -> (x/y=w5213:dbl[][])
        n3369 = Transpose 2D Array(2D array=w5295) -> (transposed array=→"Data map":dbl[][])
        n3370 = To Single Precision Float(number=w5212) -> (single precision float=w5215:sgl[][])
        n3371 = To Single Precision Float(number=w5213) -> (single precision float=w5214:sgl[][])
        n3372 = call "IMAQ ArrayToImage"("Image Pixels (Float)"=w5216, "Image"=w5252) -> ("Image Out"=w5209:T1)  [unwired: 8 in, 1 out]
        n3373 = call "IMAQ ArrayToImage"("Image Pixels (Float)"=w5211, "Image"=w5251) -> ("Image Out"=w5208:T1)  [unwired: 8 in, 1 out]
        n3374 = call "IMAQ ArrayToImage"("Image Pixels (Float)"=w5210, "Image"=w5232) -> ("Image Out"=w5207:T1)  [unwired: 8 in, 1 out]
        n3375 = call "IMAQ ArrayToImage"("Image Pixels (Float)"=w5215, "Image"=w5233) -> ("Image Out"=w5206:T1)  [unwired: 8 in, 1 out]
        n3376 = call "IMAQ ArrayToImage"("Image Pixels (Float)"=w5214, "Image"=w5234) -> ("Image Out"=w5205:T1)  [unwired: 8 in, 1 out]
        n3377 = call "IMAQ Symmetry"("Type of Symmetry"=w5204, "Image Src"=w5209) -> ("Image Dst Out"=w5202:T1)  [unwired: 3 in, 1 out]
        n3378 = call "IMAQ Symmetry"("Type of Symmetry"=w5198, "Image Src"=w5208) -> ("Image Dst Out"=w5196:T1)  [unwired: 3 in, 1 out]
        n3379 = call "IMAQ Symmetry"("Type of Symmetry"=w5194, "Image Src"=w5207) -> ("Image Dst Out"=w5192:T1)  [unwired: 3 in, 1 out]
        n3380 = call "IMAQ Symmetry"("Type of Symmetry"=w5200, "Image Src"=w5206) -> ("Image Dst Out"=→"Detection Laser X":T1)  [unwired: 3 in, 1 out]
        n3381 = call "IMAQ Symmetry"("Type of Symmetry"=w5199, "Image Src"=w5205) -> ("Image Dst Out"=→"Detection Laser Y":T1)  [unwired: 3 in, 1 out]
        n3382 = call "IMAQ Set Simple Calibration"("Calibration Axis Info"=T62 {"Origin Pixel"={"X"=0.0, "Y"=0.0}, "Angle Relative to Horizontal (deg)"=0.0, "Axis Reference"=0}, "Grid Descriptor"=T63 {"X Step"=0.3, "Y Step"=0.3, "Unit"=enum."Undefined"}, "Image"=w5196) -> ("Calibrated Image"=→"APD 2":T1)  [unwired: 7 in, 1 out]
        n3383 = call "IMAQ Set Simple Calibration"("Calibration Axis Info"=T62 {"Origin Pixel"={"X"=0.0, "Y"=0.0}, "Angle Relative to Horizontal (deg)"=0.0, "Axis Reference"=0}, "Grid Descriptor"=T63 {"X Step"=0.3, "Y Step"=0.3, "Unit"=enum."Undefined"}, "Image"=w5192) -> ("Calibrated Image"=→"APD 3":T1)  [unwired: 7 in, 1 out]
        n3384 = call "IMAQ Set Simple Calibration"("Calibration Axis Info"=T62 {"Origin Pixel"={"X"=0.0, "Y"=0.0}, "Angle Relative to Horizontal (deg)"=0.0, "Axis Reference"=0}, "Grid Descriptor"=T63 {"X Step"=0.3, "Y Step"=0.3, "Unit"=enum."Undefined"}, "Image"=w5202) -> ("Calibrated Image"=→"APD 1":T1)  [unwired: 7 in, 1 out]
      }
    }
    n3385 = case "For computing FFTs for display" shown="True" "Compute FFT" {
      tunnel: w4530 -> [_ w5505]
      frame False {
      }
      frame True {
        n3386 = Build Array("FFT 1 Choice 1", "FFT 1 Choice 2", "FFT 2 Choice 1", "FFT 2 Choice 2") -> (w5498:u16[])
        n3387 = Array Size(array=w5505) -> (size(s)=w5504:i32)
        n3388 = feedback-in #12(w5498) -> ()
        n3389 = feedback #12(u16[] [100, 100, 100, 100]) -> (w5499:u16[])
        n3390 = feedback-in #13("# Spectra to Ave.") -> ()
        n3391 = feedback #13("# Spectra to Ave.") -> (w5496:dbl)
        n3392 = Not Equal?(x="# Spectra to Ave.", y=w5496) -> (x != y?=w5495:bool)
        n3393 = Not Equal?(x=w5498, y=w5499) -> (x != y?=w5497:bool)
        n3394 = feedback #14(1.0) -> (w5482:dbl)
        n3395 = Compound Arithmetic op=OR("Reset FFT", w5497, w5495) -> (w5480:bool)
        n3396 = Select(t=1.0, s=w5480, f=w5482) -> (s? t:f=w5484:dbl)
        n3397 = Greater?(x=w5484, y="# Spectra to Ave.") -> (0:w5503:bool)
        n3398 = Increment(x=w5484) -> (x+1=w5483:dbl)
        n3399 = feedback-in #14(w5483) -> ()
        n3400 = local read "DMA Update Period (s)"() -> (w5478:dbl)
        n3401 = Multiply(x="# Spectra to Ave.", y=w5478) -> (x*y=→"Ave. Time (s)":dbl)
        n3402 = Build Array(cluster{"f0":dbl, "df":dbl, "magnitude":dbl[]} {"f0"=0.0, "df"=0.0, "magnitude"=[]} ("PSD")) -> (w5487:cluster{"f0":dbl, "df":dbl, "magnitude":dbl[]}[])
        n3403 = Build Array(w5487, w5487, w5487, w5487) -> (w5489:T72)
        n3404 = feedback #15(w5489) -> (w5494:T72)
        n3405 = for {
          N: 4 -> [_]
          tunnel: w5498 -> [w5527] mode=indexing
          tunnel: w5505 -> [w5528]
          tunnel: w5504 -> [w5530]
          tunnel: w5480 -> [w5523]
          tunnel: w5503 -> [w5522]
          tunnel: "# Spectra to Ave." -> [w5521]
          tunnel: [w5520] -> w5493 mode=indexing
          tunnel: w5494 -> [w5525] mode=indexing
          tunnel: [w5524] -> w5481 mode=indexing
          tunnel: w5484 -> [w5519]
          n3406 = Less?(x=w5527, y=w5530) -> (x < y?=w5529:bool)
          n3407 = Index Array(array=w5528, index=w5527) -> (element=w5526:waveform(dbl))
          n3408 = case shown="True" w5529 {
            tunnel: w5526 -> [_ w5547]
            tunnel: w5525 -> [w5532 w5545]
            tunnel: [w5532 w5533] -> w5524
            tunnel: w5523 -> [_ w5544]
            tunnel: w5522 -> [_ w5537]
            tunnel: w5521 -> [_ w5536]
            tunnel: [cluster{"f0":dbl, "df":dbl, "magnitude":dbl[]} {"f0"=0.0, "df"=0.0, "magnitude"=[]} ("PSD") w5538] -> w5520
            tunnel: w5519 -> [_ w5535]
            frame False {
            }
            frame True {
              n3409 = call <vilib>:"Std Deviation and Variance.vi"("X"=w5547) -> ("mean"=w5548:dbl)  [unwired: 1 in, 2 out]
              n3410 = Subtract(x=w5547, y=w5548) -> (x-y=w5546:waveform(dbl))
              n3411 = xnode "Spectral Measurements"("Signals"=w5546) -> ("PSD"=w5540:cluster{"f0":dbl, "df":dbl, "magnitude":dbl[]})  [unwired: 1 in, 1 out]
              n3412 = case shown="False" w5544 {
                tunnel: w5545 -> [w5557 _]
                tunnel: [w5553 w5562] -> w5533
                tunnel: w5540 -> [w5556 w5563]
                tunnel: w5537 -> [w5555 _]
                frame False {
                  n3413 = Build Array (concatenate)(w5557, w5556) -> (w5554:cluster{"f0":dbl, "df":dbl, "magnitude":dbl[]}[])
                  n3414 = case shown="True" w5555 {
                    tunnel: w5554 -> [w5558 w5561]
                    tunnel: [w5558 w5559] -> w5553
                    frame False {
                    }
                    frame True {
                      n3415 = Delete From Array(array=w5561, index=0) -> (array with subset deleted=w5559:cluster{"f0":dbl, "df":dbl, "magnitude":dbl[]}[])  [unwired: 1 in, 1 out]
                    }
                  }
                }
                frame True {
                  n3416 = Build Array(w5563) -> (w5562:cluster{"f0":dbl, "df":dbl, "magnitude":dbl[]}[])
                }
              }
              n3417 = for {
                tunnel: w5533 -> [w5552] mode=indexing
                tunnel: [w5551] -> w5543 mode=indexing
                workers-P: _ -> [_]
                n3418 = Unbundle By Name(w5552) -> ("magnitude"=w5551:dbl[])
              }
              n3419 = Transpose 2D Array(2D array=w5543) -> (transposed array=w5542:dbl[][])
              n3420 = for {
                tunnel: w5542 -> [w5550] mode=indexing
                tunnel: [w5549] -> w5541 mode=indexing
                workers-P: _ -> [_]
                n3421 = Add Array Elements(numeric array=w5550) -> (sum=w5549:dbl)
              }
              n3422 = Select(t=w5536, s=w5537, f=w5535) -> (s? t:f=w5534:dbl)
              n3423 = Divide(x=w5541, y=w5534) -> (x/y=w5539:dbl[])
              n3424 = Bundle By Name(cluster=w5540, "magnitude"=w5539) -> (w5538:cluster{"f0":dbl, "df":dbl, "magnitude":dbl[]})
            }
          }
        }
        n3425 = case shown="True" w5480 {
          tunnel: w5481 -> [w5512 w5518]
          tunnel: [w5512 w5513] -> w5479
          frame False {
          }
          frame True {
            n3426 = Array Subset(array=w5518, index (row)=0 ("index"), length (row)=4 ("length"), index (col)=0 ("index"), length (col)=1 ("length")) -> (w5513:T72)
          }
        }
        n3427 = feedback-in #15(w5479) -> ()
        n3428 = Split 1D Array(array=w5493, index=2) -> (first subarray=→"FFT 1":cluster{"f0":dbl, "df":dbl, "magnitude":dbl[]}[], second subarray=→"FFT 2":cluster{"f0":dbl, "df":dbl, "magnitude":dbl[]}[])
      }
    }
    n3429 = local read "Offset Values"() -> (w4569:T20)
    n3430 = local read "T1 calibration"() -> (w4611:T9)
    n3431 = local read "T2 calibration"() -> (w4610:T8)
    n3432 = call-poly <vilib>:"Index Waveform Array.vi"("index"=16, "waveform array"=w4544) -> ("waveform"=w4586:waveform(dbl))  [unwired: 8 in, 1 out]
    n3433 = Unbundle By Name(w4601) -> ("Y"=w4609:dbl[])
    n3434 = Unbundle By Name(w4598) -> ("Y"=w4608:dbl[])
    n3435 = local read "Offset file step size"() -> (w4566:dbl)
    n3436 = Unbundle By Name(w4586) -> ("Y"=→"PSD Y Sum":dbl[])
    n3437 = call "calibrate trap data V2.vi"("Offset File step size"=w4566, "delta frequency"=w4568, "Dynamic offset update"="Dynamic offset\nupdate", "Offsets"=w4569, "T2 cal"=w4610, "T2"=w4608, "T1 cal"=w4611, "T1"=w4609) -> ("T2 force (pN)"=w4602:dbl[], "T2 position (nm)"=w4603:dbl[], "T1 force (pN)"=w4604:dbl[], "T1 position (nm)"=w4605:dbl[])
    n3438 = Bundle By Name(cluster=w4601, "Y"=w4605) -> (w4600:waveform(dbl))
    n3439 = Bundle By Name(cluster=w4601, "Y"=w4604) -> (w4599:waveform(dbl))
    n3440 = Bundle By Name(cluster=w4598, "Y"=w4603) -> (w4597:waveform(dbl))
    n3441 = Bundle By Name(cluster=w4598, "Y"=w4602) -> (w4596:waveform(dbl))
    n3442 = Subtract(x=w4605, y=w4603) -> (x-y=w4766:dbl[])
    n3443 = Negate(x=w4766) -> (-x=w4649:dbl[])
    n3444 = Subtract(x=w4649, y="Offset (nm)") -> (x-y=w4752:dbl[])
    n3445 = case "Choose calibrated display" shown="2" "Calibration" {
      tunnel: w4601 -> [w5181 _ _]
      tunnel: w4598 -> [w5180 _ _]
      tunnel: [w5181 w5183 w5185] -> w4581
      tunnel: [w5180 w5182 w5184] -> w4776
      tunnel: w4600 -> [_ w5183 _]
      tunnel: w4599 -> [_ _ w5185]
      tunnel: w4597 -> [_ w5182 _]
      tunnel: w4596 -> [_ _ w5184]
      frame 0, Default {
      }
      frame 1 {
      }
      frame 2 {
      }
    }
    n3446 = Bundle By Name(cluster=w4601, "Y"=w4752) -> (w4595:waveform(dbl))
    "Bead Separation" <- w4595
    n3447 = feedback #16(w4752) -> (w4751:dbl[])
    n3448 = Build Array (concatenate)(w4752, w4751) -> (w4606:dbl[])
    n3449 = Split 1D Array(array=w4606, index=w4486) -> (first subarray=w4607:dbl[])  [unwired: 1 out]
    n3450 = feedback-in #16(w4607) -> ()
    n3451 = Build Array(w4601, w4600, w4599, w4598, w4597, w4596, w4595) -> (w4594:waveform(dbl)[])
    n3452 = Not(x="Trap Trig. Fl.") -> (.not. x?=w4671:bool)
    n3453 = Unbundle By Name(w4581) -> ("Y"=w4650:dbl[])
    n3454 = Unbundle By Name(w4776) -> ("Y"=w4753:dbl[])
    n3455 = call-poly <vilib>:"Mean.vi"("X"=w4607) -> ("mean"=w4748:dbl)  [unwired: 1 out]
    "Bead Mean (nm)" <- w4748
    n3456 = Multiply(x=w4776, y=-1.0) -> (x*y=w4577:waveform(dbl))
    n3457 = call-poly <vilib>:"Mean.vi"("X"=w4650) -> ("mean"=w4653:dbl)  [unwired: 1 out]
    "T1 X" <- w4653
